vi "XLP80_CAN_IgnoreSignals.vi"(8 "err in":errorcluster caption="error") -> (0 "err out":errorcluster caption="error")   [LabVIEW 2021]
uses:
  XLP80_Globals/XLP80_CAN_Globals.vi
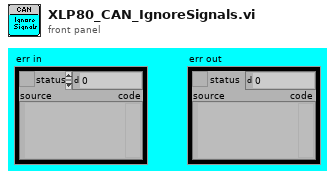
[diagram p1: front panel]
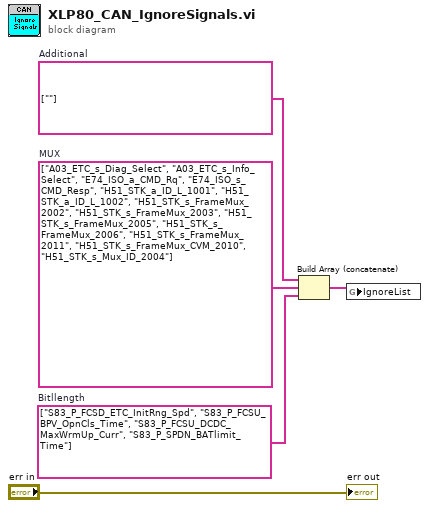
[diagram p0: block diagram]
diagram:
  w1 = string[] [""]  # Additional
  w3 = string[] ["S83_P_FCSD_ETC_InitRng_Spd", "S83_P_FCSU_BPV_OpnCls_Time", "S83_P_FCSU_DCDC_MaxWrmUp_Curr", "S83_P_SPDN_BATlimit_Time"]  # Bitllength
  w4 = string[] ["A03_ETC_s_Diag_Select", "A03_ETC_s_Info_Select", "E74_ISO_a_CMD_Rq", "E74_ISO_s_CMD_Resp", "H51_STK_a_ID_L_1001", "H51_STK_a_ID_L_1002", "H51_STK_s_FrameMux_2002", "H51_STK_s_FrameMux_2003", "H51_STK_s_FrameMux_2005", "H51_STK_s_FrameMux_2006", "H51_STK_s_FrameMux_2011", "H51_STK_s_FrameMux_CVM_2010", "H51_STK_s_Mux_ID_2004"]  # MUX
  n1 = Build Array (concatenate)(w1, w4, w3) -> (w2:string[])
  n2 = global write "XLP80_CAN_Globals.vi" "IgnoreList"(w2) -> ()
  "err out" <- "err in"
